vi "FGV_Queue.vi"(5 "Queue name":string, 7 "Queue Control":T1(ring), 8 "Error in":errorcluster, 9 "variant":variant, 10 "Message":string, 11 "queue in":refnum<queue>) -> (0 "Error out":errorcluster, 3 "queue out":refnum<queue>)   [LabVIEW 2015]
panel:
  out "element":cluster{"Message":string, "variant":variant}
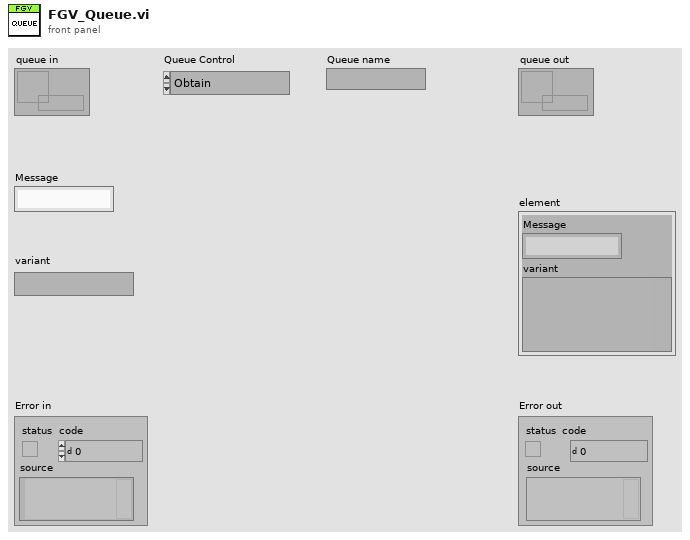
[diagram p1: front panel]
types:
  T1 = enum16{"Obtain", "Enqueue", "Enqueue (End)", "Dequeue", "Flush", "Release"}
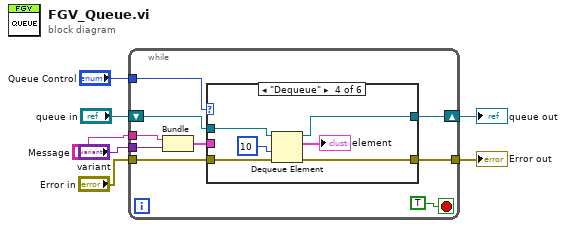
[diagram p0: block diagram]
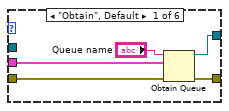
[diagram p2: hidden frame]
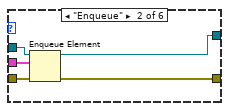
[diagram p3: hidden frame]
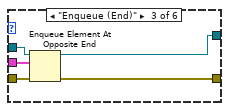
[diagram p4: hidden frame]
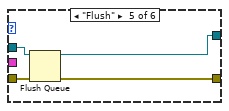
[diagram p5: hidden frame]
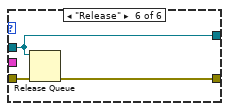
[diagram p6: hidden frame]
diagram:
  n1 = while {
    tunnel: "Queue Control" -> [w16]
    tunnel: "variant" -> [w10]
    tunnel: "Message" -> [w11]
    shift-right: [w8] -> w2
    shift-left: "queue in" -> [w13]
    tunnel: "Error in" -> [w15]
    tunnel: [w14] -> w6
    stop <- TRUE stop-if-true
    n2 = Bundle("Message"=w11, "variant"=w10) -> (w9:cluster{"Message":string, "variant":variant})  [unwired: 1 in]
    n3 = case shown="\"Dequeue\"" w16 {
      tunnel: w15 -> [w21 w23 w28 w35 w38 w43]
      tunnel: [w20 w24 w29 w34 w39 w44] -> w14
      tunnel: [w19 w25 w30 w36 w40 w42] -> w8
      tunnel: w13 -> [_ w26 w31 w37 w41 w42]
      tunnel: w9 -> [w18 w22 w27 _ _ _]
      frame "Obtain", Default {
        n4 = Obtain Queue(name (unnamed)="Queue name", element data type=w18, error in (no error)=w21) -> (queue out=w19:refnum<queue>, error out=w20:errorcluster)  [unwired: 2 in, 1 out]
      }
      frame "Enqueue" {
        n5 = Enqueue Element(queue=w26, element=w22, error in (no error)=w23) -> (queue out=w25:refnum<queue>, error out=w24:errorcluster)  [unwired: 1 in, 1 out]
      }
      frame "Enqueue (End)" {
        n6 = Enqueue Element At Opposite End(queue=w31, element=w27, error in (no error)=w28) -> (queue out=w30:refnum<queue>, error out=w29:errorcluster)  [unwired: 1 in, 1 out]
      }
      frame "Dequeue" {
        n7 = Dequeue Element(queue=w37, timeout in ms (-1)=10, error in (no error)=w35) -> (queue out=w36:refnum<queue>, element=→"element":cluster{"Message":string, "variant":variant}, error out=w34:errorcluster)  [unwired: 1 out]
      }
      frame "Flush" {
        n8 = Flush Queue(queue=w41, error in (no error)=w38) -> (queue out=w40:refnum<queue>, error out=w39:errorcluster)  [unwired: 1 out]
      }
      frame "Release" {
        n9 = Release Queue(queue=w42, error in (no error)=w43) -> (error out=w44:errorcluster)  [unwired: 1 in, 2 out]
      }
    }
  }
  "Error out" <- w6
  "queue out" <- w2
